vi "SwerveAngleEncoderConversion.vi"(11 "Voltages":dbl[](array[numeric])) -> (3 "Angles":dbl[](array[numeric]))   [LabVIEW 2018]
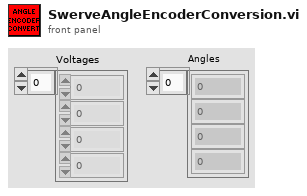
[diagram p1: front panel]
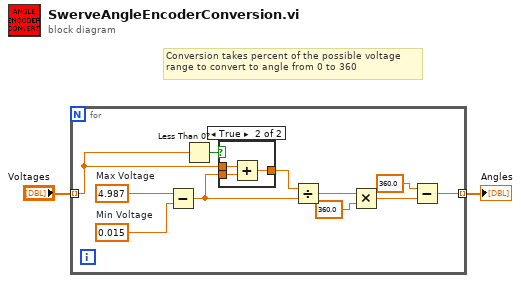
[diagram p0: block diagram]
diagram:
  # "Conversion takes percent of the possible voltage\nrange to convert to angle from 0 to 360"
  n1 = for {
    tunnel: "Voltages" -> [w13] mode=indexing
    tunnel: [w12] -> w1 mode=indexing
    w5 = 0.015  # Min Voltage
    w6 = 4.987  # Max Voltage
    n2 = Subtract(x=w6, y=w5) -> (x-y=w3:dbl)
    n3 = Less Than 0?(x=w13) -> (x < 0?=w9:bool)
    n4 = case shown="True" w9 {
      tunnel: w13 -> [w14 w17]
      tunnel: w3 -> [_ w15]
      tunnel: [w14 w16] -> w4
      frame False {
      }
      frame True {
        n5 = Add(x=w17, y=w15) -> (x+y=w16:dbl)
      }
    }
    n6 = Divide(x=w4, y=w3) -> (x/y=w11:dbl)
    n7 = Multiply(x=w11, y=360.0) -> (x*y=w7:dbl)
    n8 = Subtract(x=360.0, y=w7) -> (x-y=w12:dbl)
  }
  "Angles" <- w1
